vi "Create Log File Folder.vi"(8 "error in (no error)":errorcluster) -> (0 "error out":errorcluster, 3 "Folder Path":path)   [LabVIEW 2017, in "TestTextFileSink.lvclass"]
uses:
  TestTextFileSink.lvclass
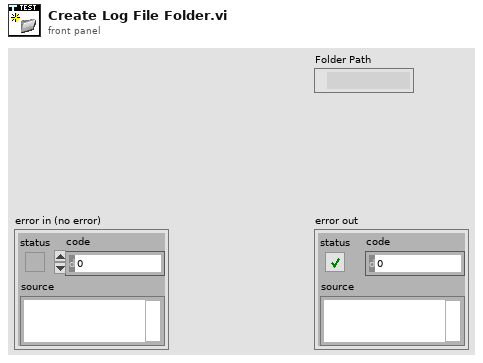
[diagram p1: front panel]
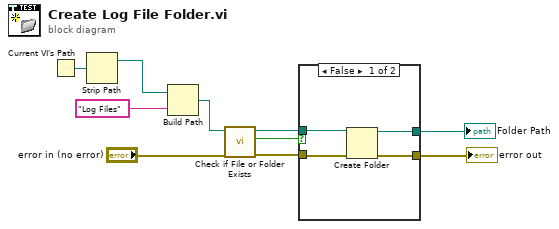
[diagram p0: block diagram]
diagram:
  n1 = Current VI's Path() -> (path=w10:path)
  n2 = Strip Path(path=w10) -> (stripped path=w9:path)  [unwired: 1 out]
  n3 = Build Path(base path=w9, name or relative path="Log Files") -> (appended path=w7:path)
  n4 = call <vilib>:"Check if File or Folder Exists.vi"("error in (no error)"="error in (no error)", "path"=w7) -> ("error out"=w4:errorcluster, "file or folder exists?"=w6:bool, "dup path"=w5:path)  [unwired: 7 in]
  n5 = case shown="False" w6 {
    tunnel: w5 -> [w14 w16]
    tunnel: w4 -> [w13 w15]
    tunnel: [w12 w16] -> w3
    tunnel: [w11 w15] -> w2
    frame False {
      n6 = Create Folder(path (use dialog)=w14, error in=w13) -> (created path=w12:path, error out=w11:errorcluster)  [unwired: 1 in, 1 out]
    }
    frame True {
    }
  }
  "Folder Path" <- w3
  "error out" <- w2
